vi "PIckPlace tester-v2.vi"() -> ()   [LabVIEW 2017]
uses:
  Shared Components/Gantry Class/Type Definitions/Virtual Modes.ctl
  Shared Components/Gantry Class/Type Definitions/Init_Modes.ctl
  Shared Components/Gantry Class/Gantry Class.lvclass
  Shared Components/Vec3d Class/Vec3d Class.lvclass
panel:
  in  "Virtual Mode":T1=enum."Virtual"
  in  "stop":bool
  out "Image":T2(plugin-control)
  out "error out":errorcluster
  in  "Config Folder":path=path "C:/Users/simra/Desktop/Research/Gantry Purdue/pixel-gantry-control/Config"
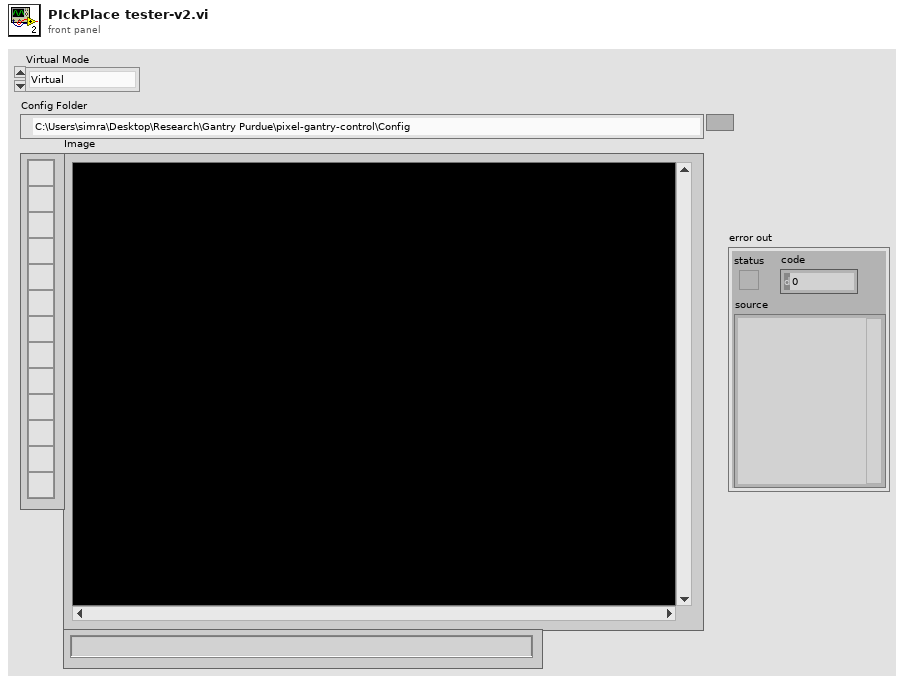
[diagram p1: front panel]
types:
  T1 = typedef "Virtual Modes.ctl" = enum16{"Nonvirtual", "Pseudovirtual", "Virtual"}
  T2 = typedef "IMAQ Image.ctl" = refnum<image>
  T3 = typedef "Init_Modes.ctl" = enum16{"Full", "Robot Only", "Dispenser Only", "Cameras Only", "Robot and Cameras", "Robot and Cameras and Dispenser", "Manifold Only"}
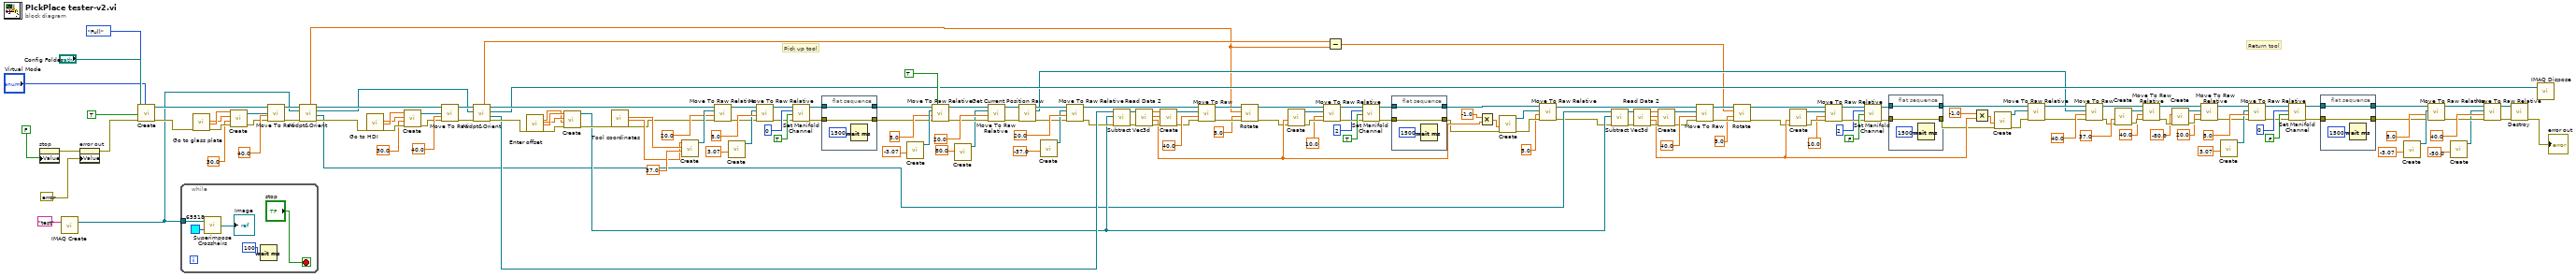
[diagram p0: block diagram]
diagram:
  # "Pick up tool"
  # "Return tool"
  n1 = property on="stop" class="Bool (strict)"("Value"=FALSE) -> (error out=w181:errorcluster)  [unwired: 2 in, 1 out]
  n2 = call "IMAQ Create"("Image Name"="test") -> ("New Image"=w77:T2)  [unwired: 4 in, 1 out]
  n3 = property on="error out" class="Clust (strict)"(error in=w181, "Value"=errorcluster {"status"=FALSE, "code"=0, "source"=""} ("error in (no error)")) -> (error out=w180:errorcluster)  [unwired: 1 in, 1 out]
  n4 = call "Create.vi"("Virtual Mode"="Virtual Mode", "error in"=w180, "HOME?"=TRUE, "Config Folder"="Config Folder", "Init Mode"=Init_Modes."Full") -> ("error out"=w177:errorcluster, "Gantry out"=w95:refnum<class "Gantry Class.lvclass">)  [unwired: 5 in]
  n5 = while {
    tunnel: w77 -> [w188]
    stop <- "stop" stop-if-true
    n6 = call "Superimpose Crosshairs.vi"("Grid Line Color"=u32 65518, "Refnum in"=w188) -> ("Refnum out"=→"Image":T2)
    n7 = Wait (ms)(milliseconds to wait=u32 100) -> ()  [unwired: 1 out]
  }
  n8 = call "Go to glass plate"("error in (no error)"=w177) -> ("Y"=w175:dbl, "X"=w176:dbl, "error out"=w173:errorcluster)  [unwired: 15 in, 1 out]
  n9 = call "Create.vi"("error in"=w173, "Z"=30.0, "Y"=w175, "X"=w176) -> ("error out"=w94:errorcluster, "Vec3d Class out"=w147:refnum<class "Vec3d Class.lvclass">)  [unwired: 6 in]
  n10 = call-dynamic "Move To Raw.vi"("error in"=w94, "Speed"=40.0, "Destination"=w147, "Gantry in"=w95) -> ("error out"=w86:errorcluster, "Gantry out"=w85:refnum<class "Gantry Class.lvclass">)  [unwired: 6 in]
  n11 = call-dynamic "Midpt&Orient.vi"("error in (no error)"=w86, "Image In"=w77, "Gantry Class in"=w85) -> ("error out"=w83:errorcluster, "Midpoint"=w29:refnum<class "Vec3d Class.lvclass">, "Image Out"=w76:T2, "Gantry Class out"=w84:refnum<class "Gantry Class.lvclass">, "Orientation"=w7:dbl)  [unwired: 4 in]
  n12 = call "Go to HDI"("error in (no error)"=w83) -> ("Y"=w92:dbl, "X"=w93:dbl, "error out"=w90:errorcluster)  [unwired: 15 in, 1 out]
  n13 = call "Create.vi"("error in"=w90, "Z"=30.0, "Y"=w92, "X"=w93) -> ("error out"=w87:errorcluster, "Vec3d Class out"=w89:refnum<class "Vec3d Class.lvclass">)  [unwired: 6 in]
  n14 = call-dynamic "Move To Raw.vi"("error in"=w87, "Speed"=40.0, "Destination"=w89, "Gantry in"=w84) -> ("error out"=w82:errorcluster, "Gantry out"=w81:refnum<class "Gantry Class.lvclass">)  [unwired: 6 in]
  n15 = call-dynamic "Midpt&Orient.vi"("error in (no error)"=w82, "Image In"=w76, "Gantry Class in"=w81) -> ("error out"=w79:errorcluster, "Midpoint"=w70:refnum<class "Vec3d Class.lvclass">, "Image Out"=w22:T2, "Gantry Class out"=w80:refnum<class "Gantry Class.lvclass">, "Orientation"=w8:dbl)  [unwired: 4 in]
  n16 = call "Enter offset"("error in (no error)"=w79) -> ("Z"=w97:dbl, "Y"=w99:dbl, "X"=w100:dbl, "error out"=w98:errorcluster)  [unwired: 14 in, 1 out]
  n17 = call "Create.vi"("error in"=w98, "Z"=w97, "Y"=w99, "X"=w100) -> ("error out"=w73:errorcluster, "Vec3d Class out"=w30:refnum<class "Vec3d Class.lvclass">)  [unwired: 6 in]
  n18 = call "Tool coordinates"("error in (no error)"=w73) -> ("Y"=w75:dbl, "X"=w74:dbl, "error out"=w72:errorcluster)  [unwired: 15 in, 1 out]
  n19 = call "Create.vi"("Z"=37.0, "Y"=w75, "X"=w74) -> ("Vec3d Class out"=w170:refnum<class "Vec3d Class.lvclass">)  [unwired: 7 in, 1 out]
  n20 = call-dynamic "Move To Raw Relative.vi"("error in"=w72, "Speed(mm/s)"=20.0, "Delta"=w170, "Gantry in"=w80) -> ("error out"=w78:errorcluster, "Gantry out"=w162:refnum<class "Gantry Class.lvclass">)  [unwired: 6 in]
  n21 = call "Create.vi"("Z"=3.07) -> ("Vec3d Class out"=w163:refnum<class "Vec3d Class.lvclass">)  [unwired: 9 in, 1 out]
  n22 = call-dynamic "Move To Raw Relative.vi"("error in"=w78, "Speed(mm/s)"=5.0, "Delta"=w163, "Gantry in"=w162) -> ("error out"=w160:errorcluster, "Gantry out"=w161:refnum<class "Gantry Class.lvclass">)  [unwired: 6 in]
  n23 = call-dynamic "Set Manifold Channel.vi"("error in"=w160, "On/Off"=TRUE, "Manifold Channel"=0, "Gantry in"=w161) -> ("error out"=w106:errorcluster, "Gantry out"=w108:refnum<class "Gantry Class.lvclass">)  [unwired: 6 in]
  n24 = flat-sequence {
    tunnel: w108 -> [w193]
    tunnel: [w193] -> w107
    tunnel: w106 -> [w191]
    tunnel: [w191] -> w105
    frame #0 {
      n25 = Wait (ms)(milliseconds to wait=u32 1500) -> ()  [unwired: 1 out]
    }
  }
  n26 = call "Create.vi"("Z"=-3.07) -> ("Vec3d Class out"=w158:refnum<class "Vec3d Class.lvclass">)  [unwired: 9 in, 1 out]
  n27 = call-dynamic "Move To Raw Relative.vi"("Wait?"=TRUE, "error in"=w105, "Speed(mm/s)"=5.0, "Delta"=w158, "Gantry in"=w107) -> ("error out"=w153:errorcluster, "Gantry out"=w154:refnum<class "Gantry Class.lvclass">)  [unwired: 5 in]
  n28 = call "Create.vi"("Y"=80.0 ("Z")) -> ("Vec3d Class out"=w152:refnum<class "Vec3d Class.lvclass">)  [unwired: 9 in, 1 out]
  n29 = call-dynamic "Move To Raw Relative.vi"("error in"=w153, "Speed(mm/s)"=20.0, "Delta"=w152, "Gantry in"=w154) -> ("error out"=w140:errorcluster, "Gantry out"=w142:refnum<class "Gantry Class.lvclass">)  [unwired: 6 in]
  n30 = call-dynamic "Get Current Position Raw.vi"("error in"=w140, "Gantry in"=w142) -> ("error out"=w139:errorcluster, "Vec3d Class out"=w16:refnum<class "Vec3d Class.lvclass">, "Gantry out"=w141:refnum<class "Gantry Class.lvclass">)  [unwired: 7 in]
  n31 = call "Create.vi"("Z"=-37.0) -> ("Vec3d Class out"=w148:refnum<class "Vec3d Class.lvclass">)  [unwired: 9 in, 1 out]
  n32 = call-dynamic "Move To Raw Relative.vi"("error in"=w139, "Speed(mm/s)"=20.0, "Delta"=w148, "Gantry in"=w141) -> ("error out"=w62:errorcluster, "Gantry out"=w60:refnum<class "Gantry Class.lvclass">)  [unwired: 6 in]
  n33 = call "Subtract Vec3d.vi"("error in (no error)"=w62, "Vec3d in 2"=w30, "Vec3d in 1"=w70) -> ("error out"=w64:errorcluster, "Vec3d Class out"=w67:refnum<class "Vec3d Class.lvclass">)  [unwired: 7 in]
  n34 = call-dynamic "Read Data 2.vi"("error in"=w64, "Vec3d in"=w67) -> ("error out"=w63:errorcluster, "Z"=w51:dbl, "Y"=w68:dbl, "X"=w69:dbl)  [unwired: 6 in]
  n35 = call "Create.vi"("error in"=w63, "Y"=w68, "X"=w69) -> ("error out"=w61:errorcluster, "Vec3d Class out"=w66:refnum<class "Vec3d Class.lvclass">)  [unwired: 7 in]
  n36 = call-dynamic "Move To Raw.vi"("error in"=w61, "Speed"=40.0, "Destination"=w66, "Gantry in"=w60) -> ("error out"=w13:errorcluster, "Gantry out"=w12:refnum<class "Gantry Class.lvclass">)  [unwired: 6 in]
  n37 = call-dynamic "Rotate.vi"("error in"=w13, "speed(deg/s)"=5.0, "distance(deg)"=w7, "Gantry in"=w12) -> ("error out"=w10:errorcluster, "Gantry out"=w11:refnum<class "Gantry Class.lvclass">)  [unwired: 6 in]
  n38 = call "Create.vi"("error in"=w10, "Z"=w51) -> ("error out"=w59:errorcluster, "Vec3d Class out"=w65:refnum<class "Vec3d Class.lvclass">)  [unwired: 8 in]
  n39 = call-dynamic "Move To Raw Relative.vi"("error in"=w59, "Speed(mm/s)"=10.0, "Delta"=w65, "Gantry in"=w11) -> ("error out"=w53:errorcluster, "Gantry out"=w54:refnum<class "Gantry Class.lvclass">)  [unwired: 6 in]
  n40 = Subtract(x=w8, y=w7) -> (x-y=w2:dbl)
  n41 = call-dynamic "Set Manifold Channel.vi"("error in"=w53, "On/Off"=TRUE, "Manifold Channel"=2, "Gantry in"=w54) -> ("error out"=w55:errorcluster, "Gantry out"=w56:refnum<class "Gantry Class.lvclass">)  [unwired: 6 in]
  n42 = flat-sequence {
    tunnel: w56 -> [w196]
    tunnel: [w196] -> w50
    tunnel: w55 -> [w194]
    tunnel: [w194] -> w49
    frame #0 {
      n43 = Wait (ms)(milliseconds to wait=u32 1500) -> ()  [unwired: 1 out]
    }
  }
  n44 = Multiply(x=-1.0, y=w51) -> (x*y=w145:dbl)
  n45 = call "Create.vi"("error in"=w49, "Z"=w145) -> ("error out"=w143:errorcluster, "Vec3d Class out"=w144:refnum<class "Vec3d Class.lvclass">)  [unwired: 8 in]
  n46 = call-dynamic "Move To Raw Relative.vi"("error in"=w143, "Speed(mm/s)"=5.0, "Delta"=w144, "Gantry in"=w50) -> ("error out"=w23:errorcluster, "Gantry out"=w24:refnum<class "Gantry Class.lvclass">)  [unwired: 6 in]
  n47 = call "Subtract Vec3d.vi"("error in (no error)"=w23, "Vec3d in 2"=w30, "Vec3d in 1"=w29) -> ("error out"=w39:errorcluster, "Vec3d Class out"=w42:refnum<class "Vec3d Class.lvclass">)  [unwired: 7 in]
  n48 = call-dynamic "Read Data 2.vi"("error in"=w39, "Vec3d in"=w42) -> ("error out"=w38:errorcluster, "Z"=w28:dbl, "Y"=w43:dbl, "X"=w44:dbl)  [unwired: 6 in]
  n49 = call "Create.vi"("error in"=w38, "Y"=w43, "X"=w44) -> ("error out"=w37:errorcluster, "Vec3d Class out"=w41:refnum<class "Vec3d Class.lvclass">)  [unwired: 7 in]
  n50 = call-dynamic "Move To Raw.vi"("error in"=w37, "Speed"=40.0, "Destination"=w41, "Gantry in"=w24) -> ("error out"=w5:errorcluster, "Gantry out"=w6:refnum<class "Gantry Class.lvclass">)  [unwired: 6 in]
  n51 = call-dynamic "Rotate.vi"("error in"=w5, "speed(deg/s)"=5.0, "distance(deg)"=w2, "Gantry in"=w6) -> ("error out"=w4:errorcluster, "Gantry out"=w3:refnum<class "Gantry Class.lvclass">)  [unwired: 6 in]
  n52 = call "Create.vi"("error in"=w4, "Z"=w28) -> ("error out"=w36:errorcluster, "Vec3d Class out"=w40:refnum<class "Vec3d Class.lvclass">)  [unwired: 8 in]
  n53 = call-dynamic "Move To Raw Relative.vi"("error in"=w36, "Speed(mm/s)"=10.0, "Delta"=w40, "Gantry in"=w3) -> ("error out"=w32:errorcluster, "Gantry out"=w33:refnum<class "Gantry Class.lvclass">)  [unwired: 6 in]
  n54 = call-dynamic "Set Manifold Channel.vi"("error in"=w32, "On/Off"=FALSE, "Manifold Channel"=2, "Gantry in"=w33) -> ("error out"=w27:errorcluster, "Gantry out"=w25:refnum<class "Gantry Class.lvclass">)  [unwired: 6 in]
  n55 = flat-sequence {
    tunnel: w25 -> [w199]
    tunnel: [w199] -> w20
    tunnel: w27 -> [w197]
    tunnel: [w197] -> w26
    frame #0 {
      n56 = Wait (ms)(milliseconds to wait=u32 1500) -> ()  [unwired: 1 out]
    }
  }
  n57 = Multiply(x=-1.0, y=w28) -> (x*y=w46:dbl)
  n58 = call "Create.vi"("error in"=w26, "Z"=w46) -> ("error out"=w21:errorcluster, "Vec3d Class out"=w17:refnum<class "Vec3d Class.lvclass">)  [unwired: 8 in]
  n59 = call-dynamic "Move To Raw Relative.vi"("error in"=w21, "Delta"=w17, "Gantry in"=w20) -> ("error out"=w18:errorcluster, "Gantry out"=w19:refnum<class "Gantry Class.lvclass">)  [unwired: 7 in]
  n60 = call-dynamic "Move To Raw.vi"("error in"=w18, "Speed"=40.0, "Destination"=w16, "Gantry in"=w19) -> ("error out"=w134:errorcluster, "Gantry out"=w137:refnum<class "Gantry Class.lvclass">)  [unwired: 6 in]
  n61 = call "Create.vi"("error in"=w134, "Z"=37.0) -> ("error out"=w133:errorcluster, "Vec3d Class out"=w136:refnum<class "Vec3d Class.lvclass">)  [unwired: 8 in]
  n62 = call-dynamic "Move To Raw Relative.vi"("error in"=w133, "Speed(mm/s)"=40.0, "Delta"=w136, "Gantry in"=w137) -> ("error out"=w128:errorcluster, "Gantry out"=w129:refnum<class "Gantry Class.lvclass">)  [unwired: 6 in]
  n63 = call "Create.vi"("error in"=w128, "Y"=-80.0) -> ("error out"=w131:errorcluster, "Vec3d Class out"=w109:refnum<class "Vec3d Class.lvclass">)  [unwired: 8 in]
  n64 = call-dynamic "Move To Raw Relative.vi"("error in"=w131, "Speed(mm/s)"=20.0, "Delta"=w109, "Gantry in"=w129) -> ("error out"=w111:errorcluster, "Gantry out"=w112:refnum<class "Gantry Class.lvclass">)  [unwired: 6 in]
  n65 = call "Create.vi"("Z"=3.07) -> ("Vec3d Class out"=w122:refnum<class "Vec3d Class.lvclass">)  [unwired: 9 in, 1 out]
  n66 = call-dynamic "Move To Raw Relative.vi"("error in"=w111, "Speed(mm/s)"=5.0, "Delta"=w122, "Gantry in"=w112) -> ("error out"=w120:errorcluster, "Gantry out"=w121:refnum<class "Gantry Class.lvclass">)  [unwired: 6 in]
  n67 = call-dynamic "Set Manifold Channel.vi"("error in"=w120, "On/Off"=FALSE, "Manifold Channel"=0, "Gantry in"=w121) -> ("error out"=w102:errorcluster, "Gantry out"=w104:refnum<class "Gantry Class.lvclass">)  [unwired: 6 in]
  n68 = flat-sequence {
    tunnel: w104 -> [w202]
    tunnel: [w202] -> w103
    tunnel: w102 -> [w200]
    tunnel: [w200] -> w101
    frame #0 {
      n69 = Wait (ms)(milliseconds to wait=u32 1500) -> ()  [unwired: 1 out]
    }
  }
  n70 = call "Create.vi"("Z"=-3.07) -> ("Vec3d Class out"=w118:refnum<class "Vec3d Class.lvclass">)  [unwired: 9 in, 1 out]
  n71 = call-dynamic "Move To Raw Relative.vi"("error in"=w101, "Speed(mm/s)"=5.0, "Delta"=w118, "Gantry in"=w103) -> ("error out"=w114:errorcluster, "Gantry out"=w115:refnum<class "Gantry Class.lvclass">)  [unwired: 6 in]
  n72 = call "Create.vi"("Z"=-50.0) -> ("Vec3d Class out"=w113:refnum<class "Vec3d Class.lvclass">)  [unwired: 9 in, 1 out]
  n73 = call-dynamic "Move To Raw Relative.vi"("error in"=w114, "Speed(mm/s)"=40.0, "Delta"=w113, "Gantry in"=w115) -> ("error out"=w15:errorcluster, "Gantry out"=w14:refnum<class "Gantry Class.lvclass">)  [unwired: 6 in]
  n74 = call "Destroy.vi"("error in"=w15, "Gantry Class in"=w14) -> ("error out"=→"error out":errorcluster)  [unwired: 9 in]
  n75 = call "IMAQ Dispose"("Image"=w22) -> ()  [unwired: 5 in, 1 out]
